vi "AppleScript Main.vi"   [LabVIEW 2018]
doc: "Main block for AppleScript.\nPut this in the autonomous vi. Do not place this inside of a loop."
panel:
  # "AppleScript\nAutonomous Scripting Language for LabVIEW\nCreated by Cory Lynch\nFRC Team 2067"
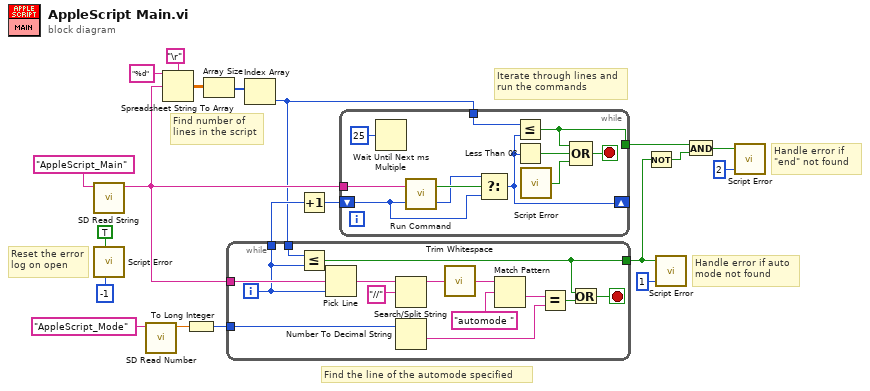
[diagram p0: block diagram]
diagram:
  # "Find number of \nlines in the script"
  # "Handle error if\n\"end\" not found"
  # "Handle error if auto\nmode not found"
  # "Iterate through lines and\nrun the commands"
  # "Find the line of the automode specified"
  # "Reset the error\nlog on open"
  n1 = call <vilib>:"SD Read String.vi"("Name"="AppleScript_Main") -> ("String"=w11:string)  [unwired: 8 in, 2 out]
  n2 = call "Script Error.vi"("Reset Log"=TRUE, "Line Number"=-1) -> ()  [unwired: 3 in, 1 out]
  n3 = call <vilib>:"SD Read Number.vi"("Name"="AppleScript_Mode") -> ("Numeric"=w17:dbl)  [unwired: 8 in, 2 out]
  n4 = Spreadsheet String To Array(delimiter (Tab)="\r", format string="%d", spreadsheet string=w11) -> (array=w15:dbl[][])  [unwired: 1 in]
  n5 = To Long Integer(number=w17) -> (32bit integer=w18:i32)
  n6 = Array Size(array=w15) -> (size(s)=w12:i32[])
  n7 = Index Array(array=w12) -> (element=w5:i32)  [unwired: 1 in]
  n8 = while {
    tunnel: w11 -> [w27]
    tunnel: w18 -> [w33]
    tunnel: [w23] -> w20
    tunnel: w5 -> [w24]
    tunnel: [w21] -> w4
    i -> [w23]
    stop <- w22 stop-if-true
    n9 = Less Or Equal?(x=w24, y=w23) -> (x <= y?=w21:bool)
    n10 = Pick Line(multi-line string=w27, line index=w23) -> (output string=w26:string)  [unwired: 1 in]
    n11 = Search/Split String(string=w26, search string/char (-)="//") -> (substring before match=w29:string)  [unwired: 1 in, 2 out]
    n12 = Number To Decimal String(number=w33) -> (decimal integer string=w31:string)  [unwired: 1 in]
    n13 = call <vilib>:"Trim Whitespace.vi"("string"=w29) -> ("trimmed string"=w28:string)  [unwired: 1 in]
    n14 = Match Pattern(string=w28, regular expression="automode ") -> (after substring=w32:string)  [unwired: 1 in, 3 out]
    n15 = Equal?(x=w32, y=w31) -> (x = y?=w25:bool)
    n16 = Or(x=w21, y=w25) -> (x .or. y?=w22:bool)
  }
  n17 = Increment(x=w20) -> (x+1=w2:i32)
  n18 = while {
    tunnel: w11 -> [w45]
    shift-right: [w42] -> _
    shift-left: w2 -> [w44]
    tunnel: w5 -> [w41]
    tunnel: [w40] -> w8
    stop <- w38 stop-if-true
    n19 = Wait Until Next ms Multiple(millisecond multiple=u32 25 ("milliseconds to wait")) -> ()  [unwired: 1 out]
    n20 = call "Run Command.vi"("Line Index In"=w44, "Script"=w45) -> ("Line Index Out"=w35:i32, "Done"=w43:bool)
    n21 = Select(t=w35, s=w43, f=w44) -> (s? t:f=w42:i32)
    n22 = Less Or Equal?(x=w41, y=w42) -> (x <= y?=w40:bool)
    n23 = Less Than 0?(x=w42) -> (x < 0?=w39:bool)
    n24 = call "Script Error.vi"() -> ("Error?"=w37:bool)  [unwired: 5 in]
    n25 = Compound Arithmetic op=OR(w40, w39, w37) -> (w38:bool)
  }
  n26 = Not(x=w4) -> (.not. x?=w7:bool)
  n27 = call "Script Error.vi"("Error?"=w4, "Error Code"=1) -> ()  [unwired: 3 in, 1 out]
  n28 = And(x=w8, y=w7) -> (x .and. y?=w6:bool)
  n29 = call "Script Error.vi"("Error?"=w6, "Error Code"=2) -> ()  [unwired: 3 in, 1 out]
